vi "IkiSetPosition.vi"(4 "Y":dbl, 5 "X":dbl, 6 "error in (no error)":errorcluster, 9 "connection ID":refnum<k5>) -> (0 "error out":errorcluster, 3 "connection ID out":refnum<k5>)   [LabVIEW 2009]
panel:
  out "Answer":string
  out "Command":string
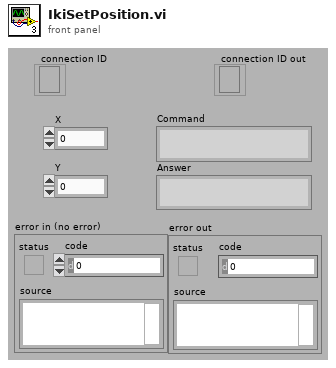
[diagram p1: front panel]
types:
  T1 = enum16{"Standard", "Buffered", "CRLF", "Immediate"}
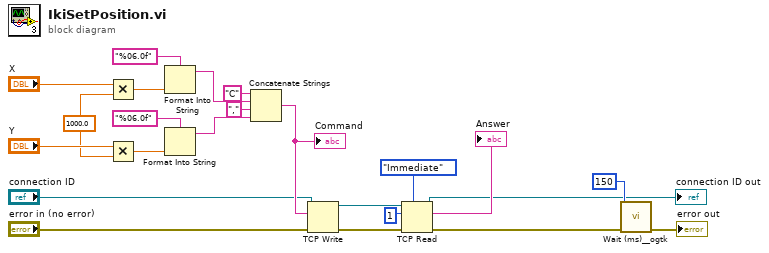
[diagram p0: block diagram]
diagram:
  w11 = 1000.0 ("y")
  n1 = Multiply(x="X", y=w11) -> (x*y=w17:dbl)
  n2 = Multiply(x="Y", y=w11) -> (x*y=w16:dbl)
  n3 = Format Into String(format string="%06.0f" ("chaîne de format"), w17) -> (resulting string=w12:string)  [unwired: 2 in, 1 out]
  n4 = Format Into String(format string="%06.0f" ("chaîne de format"), w16) -> (resulting string=w13:string)  [unwired: 2 in, 1 out]
  n5 = Concatenate Strings("C" ("chaîne"), w12, "," ("chaîne"), w13) -> (w19:string)
  "Command" <- w19
  n6 = TCP Write(connection ID="connection ID", data in=w19, error in (no error)="error in (no error)") -> (connection ID out=w4:refnum<k5>, error out=w3:errorcluster)  [unwired: 1 in, 1 out]
  n7 = TCP Read(connection ID=w4, bytes to read=1 ("octets à lire"), error in (no error)=w3, 7:T1."Immediate" ("mode (standard)")) -> (connection ID out=→"connection ID out":refnum<k5>, data out=→"Answer":string, error out=w2:errorcluster)  [unwired: 1 in]
  n8 = call <userlib>:"Wait (ms)__ogtk.vi"("error in (no error)"=w2, "milliseconds to wait"=u32 150) -> ("error out"=→"error out":errorcluster)  [unwired: 8 in, 1 out]
